vi "initialize.vi"(0 "HGF_DIMEvent":refnum<class "HGF_DIMEvent.lvclass">, 3 "initializationData":variant, 5 "error in (no error)":errorcluster, 7 "binaryString":string, 8 "I8 Array":i8[](array[numeric]), 9 "prependSize? (T)":bool, 11 "byteOrder (0:big-endian, network order)":T1(ring)) -> (14 "dup HGF_DIMEvent":refnum<class "HGF_DIMEvent.lvclass">, 17 "found?":bool, 19 "error out":errorcluster)   [LabVIEW 2012, in "HGF_DIM.lvlib" / "HGF_DIMEvent.lvclass"]
doc: "This is a dynamic dispatch VI to be implemented by child classes to initialize their attributes.\n\n<B>Recommendation:</B> Use Variant for initialization data."
uses:
  HGF_DIMEvent.lvclass
  HGF_BaseClasses/HGF_NetworkEvent/HGF_NetworkEvent.lvclass/HGF_NetworkEvent.lvclass
  HGF_DIMCommand/HGF_DIMCommand.lvclass
  HGF_DIMSubscriber/HGF_DIMSubscriber.lvclass
  HGF_DIMEvent.lvclass/HGF_DIMEvent.ctl
  DimLVEvent/LVDimInterface/LVDimInterface.dis_add_command_queue.vi
  DimLVEvent/LVDimInterface/LVDimInterface.dic_info_service_queue.vi
  DimLVEvent/LVDimInterface/LVDimInterface.lvlib
  HGF_BaseClasses/HGF_NetworkVisitor/HGF_NetworkVisitor.lvclass
  HGF_BaseClasses/HGF_Factory/HGF_Factory.lvclass
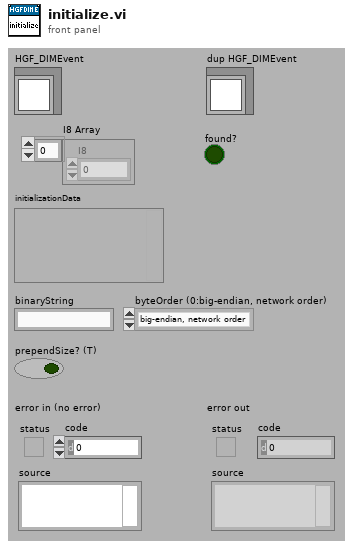
[diagram p1: front panel]
types:
  T1 = enum16{"big-endian, network order", "native, host order", "little-endian"}
  T2 = typedef "LVDimInterface.lvlib/LVDimInterface.dim service type.ctl" = u16
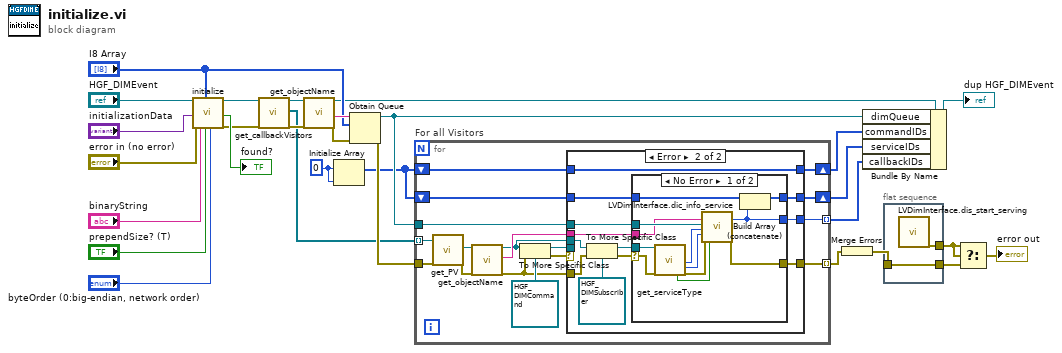
[diagram p0: block diagram]
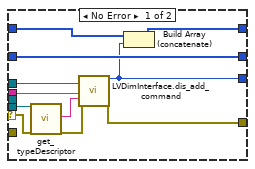
[diagram p2: hidden frame]
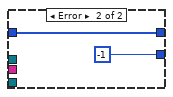
[diagram p3: hidden frame]
diagram:
  w4 = 0 ("callBackID")
  n1 = call-parent "initialize.vi"("HGF_NetworkEvent"="HGF_DIMEvent", "initializationData"="initializationData", "error in (no error)"="error in (no error)", "binaryString"="binaryString", "I8 Array"="I8 Array", "prependSize? (T)"="prependSize? (T)", "byteOrder (0:big-endian, network order)"="byteOrder (0:big-endian, network order)") -> ("dup HGF_NetworkEvent"=w17:refnum<class "HGF_DIMEvent.lvclass">, "found?"=→"found?":bool, "error out"=w15:errorcluster)  [unwired: 10 out]
  n2 = call "get_callbackVisitors.vi"("HGF_NetworkEvent"=w17, "error in (no error)"=w15) -> ("dup HGF_NetworkEvent"=w16:refnum<class "HGF_DIMEvent.lvclass">, "callbackVisitors"=w12:refnum<class "HGF_NetworkVisitor.lvclass">[], "error out"=w14:errorcluster)  [unwired: 15 out]
  n3 = call "get_objectName.vi"("HGF_Factory"=w16, "error in (no error)"=w14) -> ("dup HGF_Factory"=w19:refnum<class "HGF_DIMEvent.lvclass">, "objectName"=w24:string, "error out"=w20:errorcluster)  [unwired: 15 out]
  n4 = Initialize Array(w4, w4) -> (w3:i32[])
  n5 = Obtain Queue(name (unnamed)=w24, element data type="I8 Array", error in (no error)=w20) -> (queue out=w6:refnum<queue>, error out=w13:errorcluster)  [unwired: 2 in, 1 out]
  n6 = for "For all Visitors" {
    tunnel: w6 -> [w46]
    tunnel: w12 -> [w45] mode=indexing
    tunnel: [w37] -> w5 mode=indexing
    tunnel: w13 -> [w44]
    tunnel: [w36] -> w11 mode=indexing
    shift-right: [w32] -> w2
    shift-left: w3 -> [w33]
    shift-right: [w34] -> w1
    shift-left: w3 -> [w35]
    n7 = call "get_PV.vi"("HGF_NetworkData"=w45, "error in (no error)"=w44) -> ("HGV_PVBase"=w39:refnum<class "HGF_PVBase.lvclass">, "error out"=w40:errorcluster)  [unwired: 16 out]
    n8 = call "get_objectName.vi"("HGF_Factory"=w39, "error in (no error)"=w40) -> ("dup HGF_Factory"=w30:refnum<class "HGF_PVBase.lvclass">, "objectName"=w38:string, "error out"=w31:errorcluster)  [unwired: 15 out]
    n9 = To More Specific Class(target class=refnum<class "HGF_DIMCommand.lvclass"> refnum ("HGF_DIM.lvlib:HGF_DIMCommand.lvclass"), reference=w30, error in=w31) -> (specific class reference=w41:refnum<class "HGF_DIMCommand.lvclass">, error out=w42:errorcluster)
    n10 = case shown="Error" w42 {
      selector: w42 -> [w54 _]
      tunnel: w46 -> [w57 w69]
      tunnel: w41 -> [w55 _]
      tunnel: w38 -> [w56 w68]
      tunnel: [w49 w67] -> w37
      tunnel: [w51 w66] -> w36
      tunnel: w35 -> [w50 w63]
      tunnel: [w50 w62] -> w34
      tunnel: w33 -> [w48 w61]
      tunnel: [w47 w61] -> w32
      tunnel: w31 -> [_ w60]
      tunnel: w30 -> [_ w58]
      frame No Error {
        n11 = call "get_typeDescriptor.vi"("HGF_DIMCommand"=w55, "error in (no error)"=w54) -> ("typeDescriptor"=w53:string, "error out"=w52:errorcluster)  [unwired: 16 out]
        n12 = call-poly "LVDimInterface.dis_add_command.vi"("queueRef"=w57, "commandName"=w56, "typeDescriptor"=w53, "error in (no error)"=w52) -> ("commandID"=w49:i32, "error out"=w51:errorcluster)  [unwired: 14 out]
        n13 = Build Array (concatenate)(w48, w49) -> (w47:i32[])
      }
      frame Error {
        n14 = To More Specific Class(target class=refnum<class "HGF_DIMSubscriber.lvclass"> refnum ("HGF_DIM.lvlib:HGF_DIMServiceSubscription.lvclass"), reference=w58, error in=w60) -> (specific class reference=w64:refnum<class "HGF_DIMSubscriber.lvclass">, error out=w65:errorcluster)
        n15 = case shown="No Error" w65 {
          selector: w65 -> [w77 _]
          tunnel: w69 -> [w81 _]
          tunnel: w68 -> [w80 _]
          tunnel: [w72 -1 ("callBackID")] -> w67
          tunnel: [w79 _] -> w66
          tunnel: w64 -> [w78 _]
          tunnel: w63 -> [w71 w82]
          tunnel: [w70 w82] -> w62
          frame No Error {
            n16 = call "get_serviceType.vi"("HGF_DIMServiceInfo"=w78, "error in (no error)"=w77) -> ("stamped"=w74:bool, "timeout [s]"=w76:i32, "typeOfDimService"=w75:T2, "error out"=w73:errorcluster)  [unwired: 14 out]
            n17 = call-poly "LVDimInterface.dic_info_service.vi"("serviceName"=w80, "queueRef"=w81, "timeout [s]"=w76, "serviceType"=w75, "error in (no error)"=w73, "stamped"=w74) -> ("callBackID"=w72:i32, "error out"=w79:errorcluster)  [unwired: 12 out]
            n18 = Build Array (concatenate)(w71, w72) -> (w70:i32[])
          }
          frame Error {
          }
        }
      }
    }
  }
  n19 = Merge Errors(w11) -> (w8:errorcluster)
  n20 = Bundle By Name(cluster=w19, "dimQueue"=w6, "commandIDs"=w2, "serviceIDs"=w1, "callbackIDs"=w5) -> (→"dup HGF_DIMEvent":refnum<class "HGF_DIMEvent.lvclass">)
  n21 = flat-sequence {
    tunnel: [w85] -> w9
    tunnel: w8 -> [w84]
    tunnel: [w84] -> w7
    frame #0 {
      n22 = call "LVDimInterface.dis_start_serving.vi"() -> ("error out"=w85:errorcluster)  [unwired: 2 in, 17 out]
    }
  }
  n23 = Select(t=w9, s=w9, f=w7) -> (s? t:f=→"error out":errorcluster)
